vi "SubVI_Circle_element_Auto #.vi"(8 "Error In":errorcluster, 10 "Parameter_Circle":T1={"ROI Descriptor"={"Global Rectangle"=[], "Contours"=[]}, "Edge Options"={"Edge Options"={"Edge Polarity"=0, "Kernel Size"=3, "Width"=3, "Minimum Edge Strength"=10.0, "Interpolation Type"=enum."Bilinear Fixed", "Data Processing Method"=enum."Average"}, "Step Size"=3.0, "Scan Direction"=0, "Auto"=FALSE, "SD"=0.0}, "條件"={"半徑最大值"=0.0, "半徑最小值"=5.0}} {"Edge Options"."Scan Direction" items=["Outside To Inside", "Inside To Outside"]; "Edge Options"."Edge Options"."Edge Polarity" items=["All Edges", "Rising Edges", "Falling Edges"]; "Edge Options"."Edge Options"."Minimum Edge Strength" format="%.2f"; "Edge Options"."Edge Options"."Width" step=2; "Edge Options"."Edge Options"."Kernel Size" step=2; "ROI Descriptor"."Contours"."Type" items=["No Selection", "Point", "Line", "Rectangle", "Oval", "Polygon", "Free", "Annulus", "Unused2", "Unused3", "Broken Line", "Free Hand Line", "Rotated Rectangle"]}, 11 "Image In":T4) -> (0 "Error Out":errorcluster, 2 "Location":cluster{"X":sgl, "Y":sgl}[](array[cluster]) {"Y" format="%.2g"; "X" format="%.2f"}, 3 "Image Out":T4)   [LabVIEW 2013]
uses:
  <vilib>/vision/Image Controls.llb/IMAQ Image.ctl
  Control/Control Find Circle #2.ctl
  <vilib>/vision/Measure.llb/Edge Options.ctl
  <vilib>/vision/Measure.llb/Edge Polarity.ctl
  <vilib>/vision/NI_Vision_Development_Module.lvlib
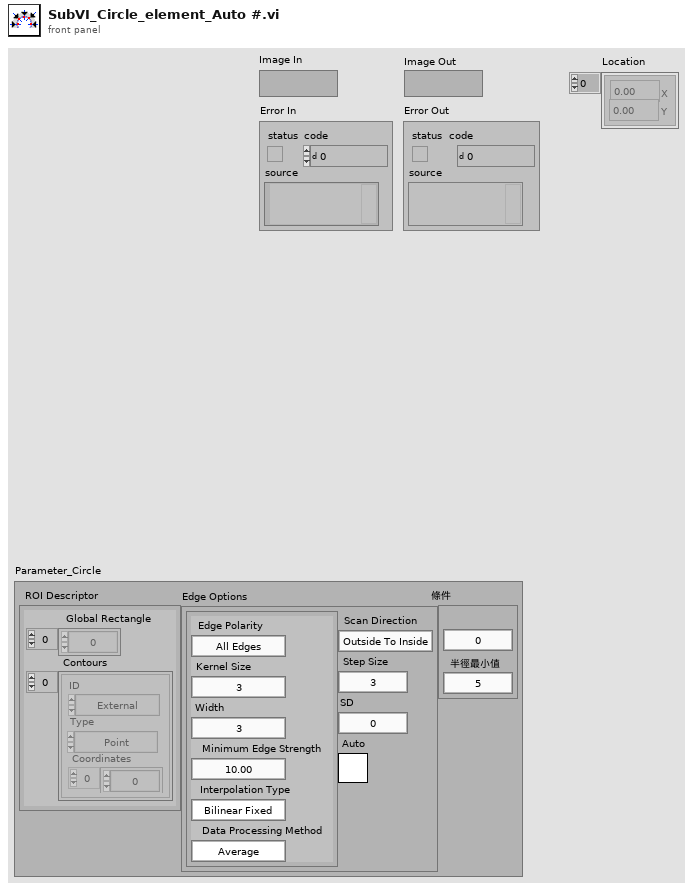
[diagram p1: front panel]
types:
  T1 = typedef "Control Find Circle #2.ctl" = cluster{"ROI Descriptor":cluster{"Global Rectangle":i32[], "Contours":cluster{"ID":enum32{"External", "Internal"}, "Type":u32, "Coordinates":i32[]}[]}, "Edge Options":cluster{"Edge Options":T2, "Step Size":dbl, "Scan Direction":u16, "Auto":bool, "SD":dbl}, "條件":cluster{"半徑最大值":dbl, "半徑最小值":dbl}}
  T2 = typedef "Edge Options.ctl" = cluster{"Edge Polarity":T3, "Kernel Size":u32, "Width":u32, "Minimum Edge Strength":sgl, "Interpolation Type":enum32{"Zero Order", "Bilinear", "Quadratic", "Cubic", "Bilinear Fixed"}, "Data Processing Method":enum32{"Average", "Median"}}
  T3 = typedef "Edge Polarity.ctl" = u32
  T4 = typedef "IMAQ Image.ctl" = refnum<image>
  T5 = typedef "ROI Descriptor" = cluster{"Global Rectangle":i32[], "Contours":cluster{"ID":enum32{"External", "Internal"}, "Type":u32, "Coordinates":i32[]}[]}
  T6 = cluster{"ID":enum32{"External", "Internal"}, "Type":u32, "Coordinates":i32[]}
  T7 = enum16{"Get First Edge", "Get First + Last Edge", "Get All Edges", "Get Best Edge"}
  T8 = cluster{"Global Rectangle":i32[], "Contours":cluster{"ID":enum32{"External", "Internal"}, "Type":u32, "Coordinates":i32[]}[]}
  T9 = typedef "Search Line.ctl" = cluster{"Start Point":cluster{"X":sgl, "Y":sgl}, "End Point":cluster{"X":sgl, "Y":sgl}, "Edge Info":T10[], "Edge Map":dbl[], "Calibration Valid":bool}
  T10 = typedef "Edge New.ctl" = cluster{"Location (Pixel)":cluster{"X":sgl, "Y":sgl}, "Location (Real-World)":cluster{"X":sgl, "Y":sgl}, "Distance (Pixel)":dbl, "Distance (Real-World)":dbl, "Strength":dbl, "Noise":dbl, "Rising?":bool}
  T11 = cluster{"ID":enum32{"External", "Internal"}, "Type":u32, "Coordinates":i32[]}[]
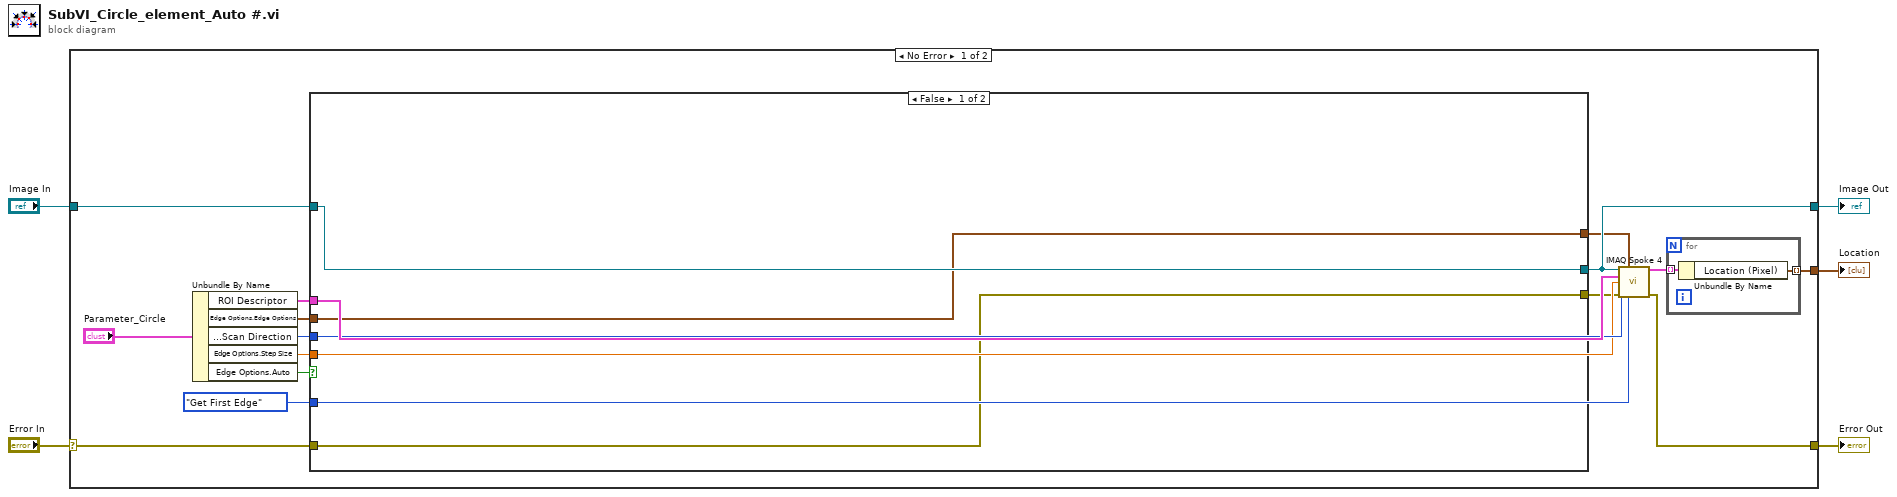
[diagram p0: block diagram]
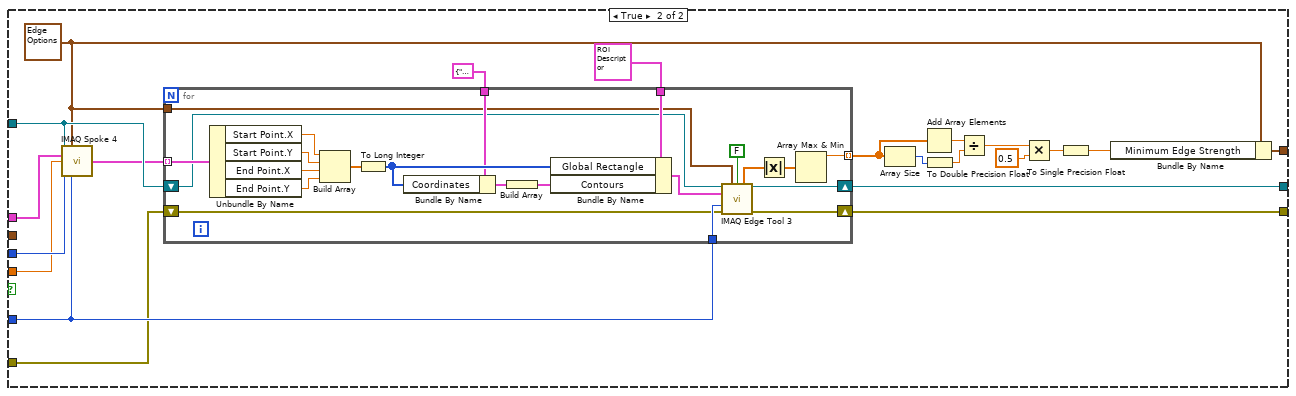
[diagram p2: hidden frame]
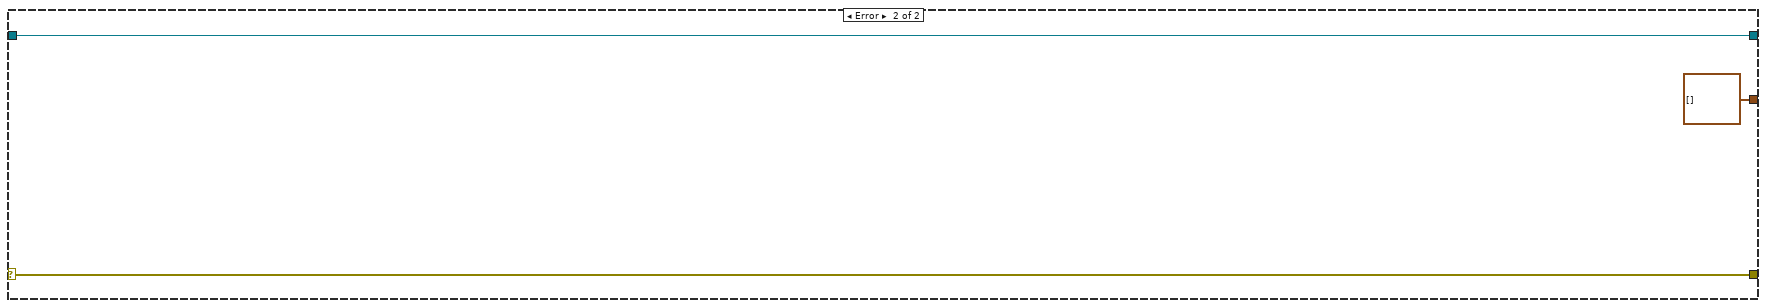
[diagram p3: hidden frame]
diagram:
  n1 = case shown="No Error" "Error In" {
    selector: "Error In" -> [w7 w70]
    tunnel: [w20 cluster{"X":sgl, "Y":sgl}[] []] -> w5
    tunnel: [w19 w70] -> w4
    tunnel: "Image In" -> [w18 w71]
    tunnel: [w17 w71] -> w2
    frame No Error {
      w9 = T7."Get First Edge" ("Process")
      n2 = Unbundle By Name("Parameter_Circle") -> ("ROI Descriptor"=w15:T8, "Edge Options.Edge Options"=w12:T2, "Edge Options.Scan Direction"=w14:u16, "Edge Options.Step Size"=w13:dbl, "Edge Options.Auto"=w6:bool)
      n3 = case shown="False" w6 {
        tunnel: w18 -> [w23 w44]
        tunnel: [w23 w43] -> w17
        tunnel: w15 -> [_ w42]
        tunnel: w14 -> [_ w41]
        tunnel: w13 -> [_ w40]
        tunnel: w12 -> [w22 _]
        tunnel: [w22 w28] -> w11
        tunnel: [w21 w27] -> w10
        tunnel: w9 -> [_ w26]
        tunnel: w7 -> [w21 w25]
        frame False {
        }
        frame True {
          w24 = T2 {"Edge Polarity"=0, "Kernel Size"=3, "Width"=3, "Minimum Edge Strength"=10.0, "Interpolation Type"=enum."Bilinear Fixed", "Data Processing Method"=enum."Average"} ("Edge Options")
          n4 = call "IMAQ Spoke 4"("Image"=w44, "Edge Options"=w24, "ROI Descriptor"=w42, "Step Size"=w40, "Scan Direction"=w41, "Process"=w26) -> ("Search Lines"=w39:T9[])  [unwired: 6 in, 3 out]
          n5 = for {
            tunnel: w39 -> [w66] mode=indexing
            tunnel: w26 -> [w58]
            tunnel: T5 {"Global Rectangle"=[0, 0, 0, 0], "Contours"=[{"ID"=enum."External", "Type"=2, "Coordinates"=[0, 0, 0, 0]}]} ("ROI Descriptor") -> [w56]
            tunnel: T6 {"ID"=enum."External", "Type"=2, "Coordinates"=[0, 0, 0, 0]} -> [w57]
            tunnel: w24 -> [w55]
            shift-right: [w48] -> w43
            shift-left: w44 -> [w47]
            tunnel: [w54] -> w29 mode=indexing
            shift-right: [w45] -> w27
            shift-left: w25 -> [w46]
            n6 = Unbundle By Name(w66) -> ("Start Point.X"=w65:sgl, "Start Point.Y"=w64:sgl, "End Point.X"=w63:sgl, "End Point.Y"=w62:sgl)
            n7 = Build Array(w65, w64, w63, w62) -> (w61:sgl[])
            n8 = To Long Integer(number=w61) -> (32bit integer=w59:i32[])
            n9 = Bundle By Name(cluster=w57, "Coordinates"=w59) -> (w60:T6)
            n10 = Build Array(w60) -> (w52:T11)
            n11 = Bundle By Name(cluster=w56, "Global Rectangle"=w59, "Contours"=w52) -> (w51:T5)
            n12 = call "IMAQ Edge Tool 3"("Image"=w47, "Edge Options"=w55, "Optimized Mode"=FALSE, "ROI Descriptor"=w51, "Process"=w58, "error in (no error)"=w46) -> ("Image (duplicate)"=w48:T4, "Gradient Values"=w49:dbl[], "error out"=w45:errorcluster)  [unwired: 5 in, 2 out]
            n13 = Absolute Value(x=w49) -> (abs(x)=w50:dbl[])
            n14 = Array Max & Min(array=w50) -> (max value=w54:dbl)  [unwired: 3 out]
          }
          n15 = Array Size(array=w29) -> (size(s)=w34:i32)
          n16 = Add Array Elements(numeric array=w29) -> (sum=w30:dbl)
          n17 = To Double Precision Float(number=w34) -> (double precision float=w31:dbl)
          n18 = Divide(x=w30, y=w31) -> (x/y=w32:dbl)
          n19 = Multiply(x=w32, y=0.5) -> (x*y=w35:dbl)
          n20 = To Single Precision Float(number=w35) -> (single precision float=w36:sgl)
          n21 = Bundle By Name(cluster=w24, "Minimum Edge Strength"=w36) -> (w28:T2)
        }
      }
      n22 = call "IMAQ Spoke 4"("Image"=w17, "Edge Options"=w11, "ROI Descriptor"=w15, "Step Size"=w13, "Scan Direction"=w14, "error in (no error)"=w10, "Process"=w9) -> ("First Edges"=w8:T10[], "error out"=w19:errorcluster)  [unwired: 5 in, 2 out]
      n23 = for {
        tunnel: w8 -> [w68] mode=indexing
        tunnel: [w67] -> w20 mode=indexing
        n24 = Unbundle By Name(w68) -> ("Location (Pixel)"=w67:cluster{"X":sgl, "Y":sgl})
      }
    }
    frame Error {
    }
  }
  "Location" <- w5
  "Error Out" <- w4
  "Image Out" <- w2
